vi "Error Handling Example.vi"() -> ()   [LabVIEW 2015]
uses:
  <vilib>/DAQmx/create/channels.llb/DAQmx Create Channel (AI-Acceleration-Accelerometer).vi
  <vilib>/DAQmx/configure/timing.llb/DAQmx Timing (Sample Clock).vi
  <vilib>/DAQmx/read.llb/DAQmx Read (Analog 1D DBL 1Chan NSamp).vi
panel:
  out "Acceleration Data - Graph":dbl[](graph)
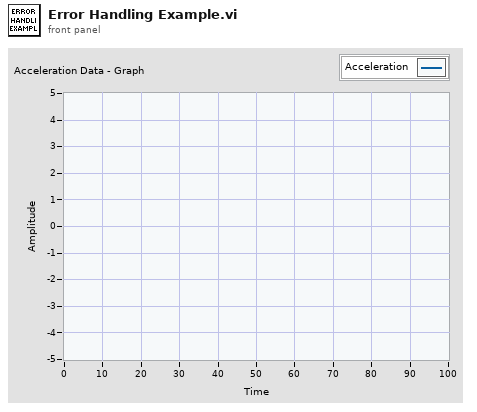
[diagram p1: front panel]
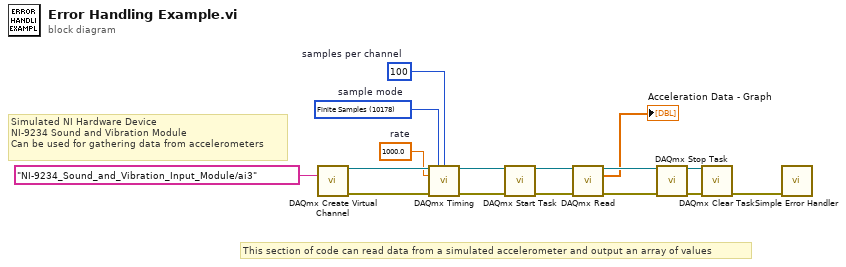
[diagram p0: block diagram]
diagram:
  w3 = 1000.0  # rate
  w4 = 100  # samples per channel
  w5 = 10178 items=["Finite Samples"=10178, "Continuous Samples"=10123, "Hardware Timed Single Point"=12522]  # sample mode
  # "This section of code can read data from a simulated accelerometer and output an array of values"
  # "Simulated NI Hardware Device\nNI-9234 Sound and Vibration Module\nCan be used for gathering data from accelerometers"
  n1 = call-poly <vilib>:"DAQmx Create Virtual Channel.vi"("physical channels"=tag "NI-9234_Sound_and_Vibration_Input_Module/ai3") -> ("task out"=w9:refnum<k21>, "error out"=w8:errorcluster)  [unwired: 13 in]
  n2 = call-poly <vilib>:"DAQmx Timing.vi"("task/channels in"=w9, "sample mode"=w5, "samples per channel"=w4, "rate"=w3, "error in"=w8) -> ("task out"=w7:refnum<k21>, "error out"=w6:errorcluster)  [unwired: 9 in]
  n3 = call <vilib>:"DAQmx Start Task.vi"("task/channels in"=w7, "error in"=w6) -> ("task out"=w15:refnum<k21>, "error out"=w16:errorcluster)  [unwired: 12 in]
  n4 = call-poly <vilib>:"DAQmx Read.vi"("task/channels in"=w15, "error in"=w16) -> ("task out"=w13:refnum<k21>, "data"=→"Acceleration Data - Graph":dbl[], "error out"=w12:errorcluster)  [unwired: 11 in]
  n5 = call <vilib>:"DAQmx Stop Task.vi"("task/channels in"=w13, "error in"=w12) -> ("task out"=w14:refnum<k21>, "error out"=w11:errorcluster)  [unwired: 12 in]
  n6 = call <vilib>:"DAQmx Clear Task.vi"("task in"=w14, "error in"=w11) -> ("error out"=w1:errorcluster)  [unwired: 13 in]
  n7 = call <vilib>:"Simple Error Handler.vi"("error in (no error)"=w1) -> ()  [unwired: 4 in, 5 out]
